vi "Configure Mask Test.vi"(0 "VISA resource name":refnum<visa-resource-name>, 1 "Enable Mask Test (Enable)":bool=TRUE, 5 "Source (1: Channel 1)":i32(ring)=1 items=["Channel 1"=1, "Channel 2"=2, "Channel 3"=3, "Channel 4"=4, "Function 1"=5, "Function 2"=6, "Function 3"=7, "Function 4"=8], 7 "Trigger Source (1: Channel 1)":i32(ring)=1 items=["Channel 1"=1, "Channel 2"=2, "Channel 3"=3, "Channel 4"=4], 9 "Impedance (0: None)":i32(ring) items=["None", "IMP75", "IMP100", "IMP110", "IMP120"], 11 "error in (no error)":errorcluster, 12 "Run":T2={"Enable Stop on Fail (Disable)"=FALSE, "Run Mode (0: Forever)"=0, "Waveform Count (1000)"=1000, "Time (1.0 min)"=1.0} {"Time (1.0 min)" format="%#.1g"; "Run Mode (0: Forever)" items=["Forever", "Waveform", "Time"]}, 13 "Test Options":T3={"Enable Averaging (Disable)"=FALSE, "Average Count (16)"=16, "Enable Use File Setup (Enable)"=TRUE}, 14 "Pulse Amplitude":T1={"Maximum Amplitude (V)"=1.0, "Minimum Amplitude (V)"=1.0}) -> (4 "VISA resource name out":refnum<visa-resource-name>, 15 "error out":errorcluster)   [LabVIEW 2012, in "Agilent 8000 Series.lvlib"]
doc: "Configures the Mask test and the parameters required for a mask test. This VI has to be called before calling any other Mask related VIs."
uses:
  Agilent 8000 Series.lvlib
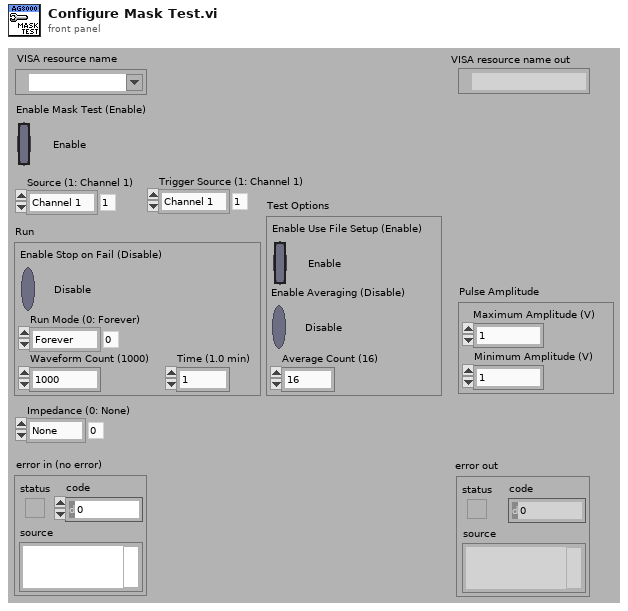
[diagram p1: front panel]
types:
  T1 = cluster{"Maximum Amplitude (V)":dbl, "Minimum Amplitude (V)":dbl}
  T2 = cluster{"Enable Stop on Fail (Disable)":bool, "Run Mode (0: Forever)":i32, "Waveform Count (1000)":u32, "Time (1.0 min)":dbl}
  T3 = cluster{"Enable Averaging (Disable)":bool, "Average Count (16)":u32, "Enable Use File Setup (Enable)":bool}
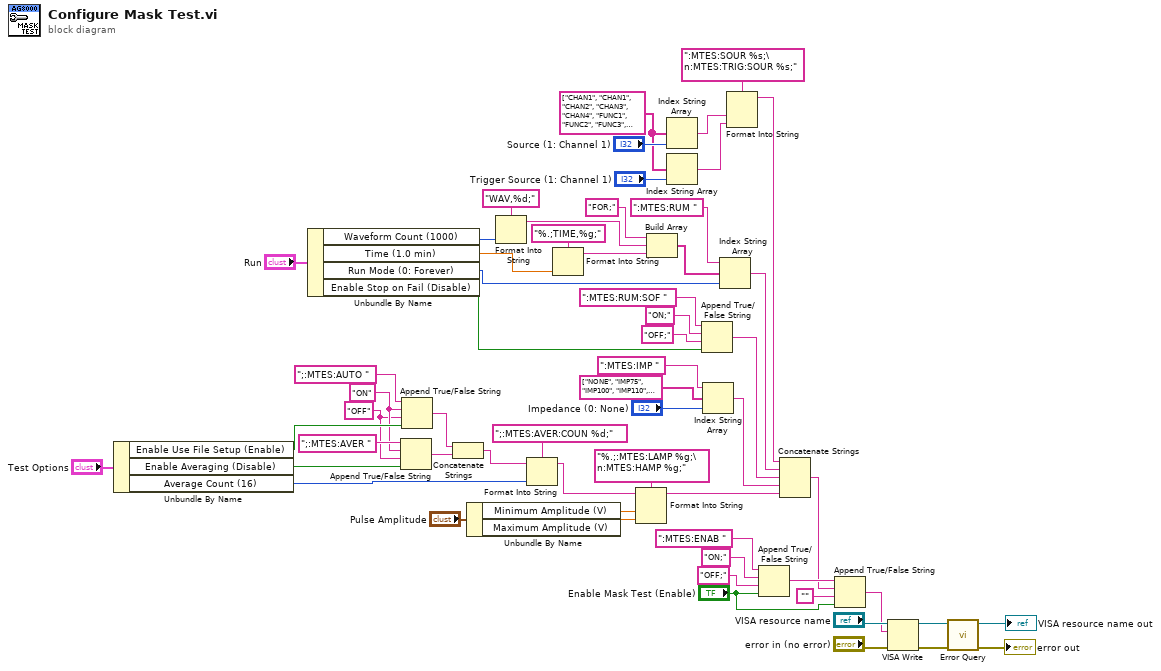
[diagram p0: block diagram]
diagram:
  w1 = "OFF" ("false string")
  w2 = "ON" ("true string")
  w48 = string[] ["CHAN1", "CHAN1", "CHAN2", "CHAN3", "CHAN4", "FUNC1", "FUNC2", "FUNC3", "FUNC4", "WMEM1", "WMEM2", "WMEM3", "WMEM4", "DIG0", "DIG1", "DIG2", "DIG3", "DIG4", "DIG5", "DIG6", "DIG7", "DIG8", "DIG9", "DIG10", "DIG11", "DIG12", "DIG13", "DIG14", "DIG15", "AUX", "LINE"]
  n1 = Unbundle By Name("Test Options") -> ("Enable Use File Setup (Enable)"=w6:bool, "Enable Averaging (Disable)"=w27:bool, "Average Count (16)"=w28:u32)
  n2 = Unbundle By Name("Run") -> ("Waveform Count (1000)"=w45:u32, "Time (1.0 min)"=w43:dbl, "Run Mode (0: Forever)"=w37:i32, "Enable Stop on Fail (Disable)"=w35:bool)
  n3 = Append True/False String(1:w27, 2:w1, 3:w2, 4:";:MTES:AVER " ("string (\"\")")) -> (0:w3:string)
  n4 = Append True/False String(1:w6, 2:w1, 3:w2, 4:";:MTES:AUTO " ("string (\"\")")) -> (0:w5:string)
  n5 = Concatenate Strings(w5, w3) -> (w4:string)
  n6 = Unbundle By Name("Pulse Amplitude") -> ("Minimum Amplitude (V)"=w25:dbl, "Maximum Amplitude (V)"=w24:dbl)
  n7 = Format Into String(format string="WAV,%d;", w45) -> (resulting string=w40:string)  [unwired: 2 in, 1 out]
  n8 = Format Into String(format string=";:MTES:AVER:COUN %d;", initial string=w4, w28) -> (resulting string=w20:string)  [unwired: 1 in, 1 out]
  n9 = Format Into String(format string="%.;TIME,%g;", w43) -> (resulting string=w42:string)  [unwired: 2 in, 1 out]
  n10 = Format Into String(format string="%.;:MTES:LAMP %g;\n:MTES:HAMP %g;", initial string=w20, w25, w24) -> (resulting string=w18:string)  [unwired: 1 in, 1 out]
  n11 = Build Array("FOR;", w40, w42) -> (w38:string[])
  n12 = Index String Array(1:"Source (1: Channel 1)", 2:w48) -> (0:w51:string)  [unwired: 1 in]
  n13 = Index String Array(1:"Trigger Source (1: Channel 1)", 2:w48) -> (0:w47:string)  [unwired: 1 in]
  n14 = Append True/False String(1:w35, 2:"OFF;" ("false string"), 3:"ON;" ("true string"), 4:":MTES:RUM:SOF " ("string (\"\")")) -> (0:w19:string)
  n15 = Index String Array(1:"Impedance (0: None)", 2:string[] ["NONE", "IMP75", "IMP100", "IMP110", "IMP120"] ("string array"), 3:":MTES:IMP " ("string (\"\")")) -> (0:w14:string)
  n16 = Index String Array(1:w37, 2:w38, 3:":MTES:RUM " ("string (\"\")")) -> (0:w21:string)
  n17 = Format Into String(format string=":MTES:SOUR %s;\n:MTES:TRIG:SOUR %s;", w51, w47) -> (resulting string=w22:string)  [unwired: 2 in, 1 out]
  n18 = Append True/False String(1:"Enable Mask Test (Enable)", 2:"OFF;" ("false string"), 3:"ON;" ("true string"), 4:":MTES:ENAB " ("string (\"\")")) -> (0:w11:string)
  n19 = Concatenate Strings(w22, w21, w19, w14, w18) -> (w10:string)
  n20 = Append True/False String(1:"Enable Mask Test (Enable)", 2:"", 3:w10, 4:w11) -> (0:w9:string)
  n21 = VISA Write(VISA resource name="VISA resource name", write buffer=w9, error in (no error)="error in (no error)") -> (VISA resource name out=w58:refnum<visa-resource-name>, error out=w57:errorcluster)  [unwired: 1 out]
  n22 = call "Error Query.vi"("error in (no error)"=w57, "VISA resource name"=w58) -> ("error out"=→"error out":errorcluster, "VISA resource name out"=→"VISA resource name out":refnum<visa-resource-name>)  [unwired: 6 in, 2 out]
